vi "[FPGA] Zero Crossing with Debounce Float Multichannel.vi"(0 "input":sgl, 1 "reset":bool, 5 "Channel #":u32, 7 "direction":enum8{"either", "minus-plus", "plus-minus"}(ring), 9 "Debounce (iterations)":i32=1) -> (4 "crossing":bool)   [LabVIEW 2015]
doc: "Detects zero crossings of an input signal. The data type you wire to <B>input</B> determines the <B>output</B> data type."
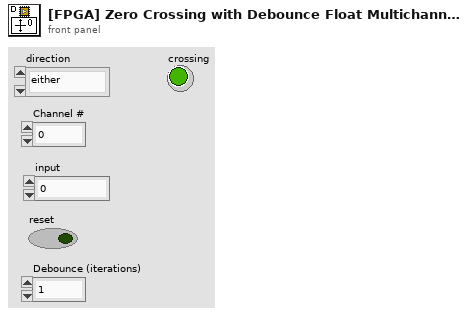
[diagram p1: front panel]
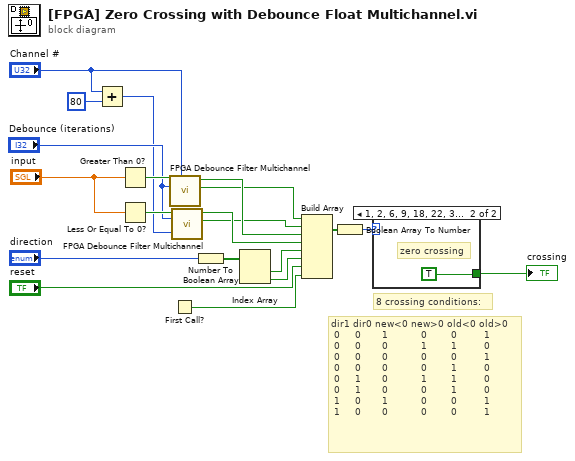
[diagram p0: block diagram]
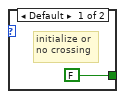
[diagram p2: hidden frame]
diagram:
  # "8 crossing conditions:"
  # "dir1 dir0 new<0 new>0 old<0 old>0\n 0     0       1           0        0         1\n 0     0       0           1        1         0\n 0     0       0           0        0         1\n 0     0       0           0        1         0\n 0     1       0           1        1         0\n 0     1       0           0        1         0\n 1     0       1           0        0         1\n 1     0       0           0        0         1"
  n1 = Add(x="Channel #", y=u32 80) -> (x+y=w3:u32)
  n2 = Greater Than 0?(x="input") -> (x > 0?=w10:bool)
  n3 = Less Or Equal To 0?(x="input") -> (x <= 0?=w8:bool)
  n4 = call "FPGA Debounce Filter Multichannel.vi"("Channel #"="Channel #", "Debounce (iterations)"="Debounce (iterations)", "Input"=w10) -> ("Output[k-1]"=w2:bool, "Output"=w9:bool)  [unwired: 5 in]
  n5 = First Call?() -> (First Call?: T/F=w14:bool)
  n6 = call "FPGA Debounce Filter Multichannel.vi"("Channel #"=w3, "Debounce (iterations)"="Debounce (iterations)", "Input"=w8) -> ("Output[k-1]"=w1:bool, "Output"=w7:bool)  [unwired: 5 in]
  n7 = Number To Boolean Array(number="direction") -> (Boolean array=w12:bool[])
  n8 = Index Array(array=w12) -> (element #1=w13:bool, element #2=w16:bool)  [unwired: 2 in]
  n9 = Build Array(w2, w1, w9, w7, w13, w16, "reset", w14) -> (w11:bool[])
  n10 = Boolean Array To Number(Boolean array=w11) -> (number=w15:u8)
  n11 = case shown="1, 2, 6, 9, 18, 22, 33, 41" w15 {
    tunnel: [FALSE TRUE] -> w17
    frame Default {
      # "initialize or\nno crossing"
    }
    frame 1, 2, 6, 9, 18, 22, 33, 41 {
      # "zero crossing"
    }
  }
  "crossing" <- w17
